vi "Read State.vi"(8 "error in (no error)":errorcluster, 11 "B Context State in":refnum<class "B Context State.lvclass">) -> (0 "error out":errorcluster, 2 "State":refnum<class "State Pattern.lvclass">, 3 "B Context State out":refnum<class "B Context State.lvclass">)   [LabVIEW 2021, in "Context.lvlib" / "B Context State.lvclass"]
uses:
  B Context State.lvclass
  State Pattern/State Pattern/State Pattern.lvclass
  B Context State.lvclass/B Context State.ctl
  Context/Context.lvclass
  C:/PPLs/Design-Patterns/State Pattern/State Pattern/State Pattern.lvclass
  C:/Program Files/National Instruments/LabVIEW 2021/vi.lib/ActorFramework/Actor/Actor.lvclass
  C:/PPLs/Design-Patterns/State Pattern/State Pattern/State Change Core/State Change Core/State Change Core.lvclass
  C:/PPLs/Design-Patterns/State Pattern/State P/State Pattern/State Pattern.lvclass
  C:/PPLs/Design-Patterns/State Pattern/Context/Context State/Context State.lvclass
  C:/PPLs/Design-Patterns/State Pattern/Context/Context/Context.lvclass
  C:/PPLs/Design-Patterns/State Pattern/Flip States/Flip States/Flip States.lvclass
  C:/PPLs/Design-Patterns/State Pattern/xxxx/xxxx/xxxx.lvclass
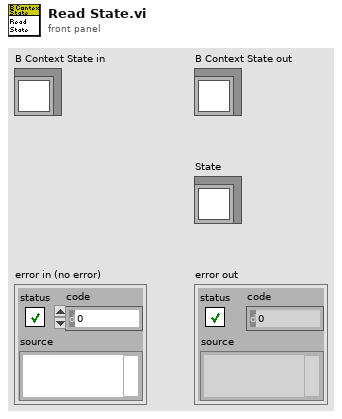
[diagram p1: front panel]
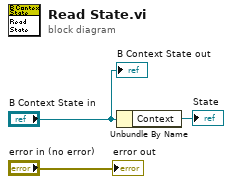
[diagram p0: block diagram]
diagram:
  n1 = Unbundle By Name("B Context State in") -> ("Context"=→"State":refnum<class "Context.lvclass">)
  "error out" <- "error in (no error)"
  "B Context State out" <- "B Context State in"
